vi "Main.vi"() -> ()   [LabVIEW 2014]
uses:
  Electrical/Electrical.lvclass
  White/White.lvclass
  Petrol/Petrol.lvclass
  Black/Black.lvclass
panel:
  out "MsgString":string
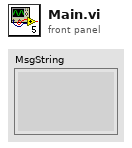
[diagram p1: front panel]
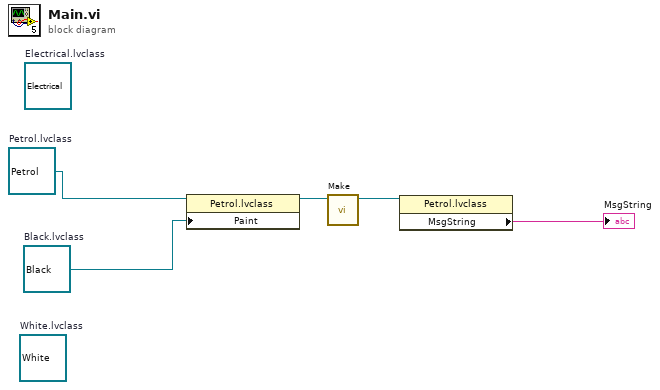
[diagram p0: block diagram]
diagram:
  w2 = refnum<class "Black.lvclass"> refnum  # Black.lvclass
  w1 = refnum<class "Petrol.lvclass"> refnum  # Petrol.lvclass
  (unwired) refnum<class "White.lvclass"> refnum  # White.lvclass
  (unwired) refnum<class "Electrical.lvclass"> refnum  # Electrical.lvclass
  n1 = property class="Petrol.lvclass"(reference=w1, "Paint"=w2) -> (reference out=w3:refnum<class "Petrol.lvclass">)  [unwired: 1 in, 1 out]
  n2 = call-dynamic "Make.vi"("Electrical in"=w3) -> ("Electrical out"=w5:refnum<class "Petrol.lvclass">)  [unwired: 9 in, 1 out]
  n3 = property class="Petrol.lvclass"(reference=w5) -> ("MsgString"=→"MsgString":string)  [unwired: 1 in, 2 out]
